vi "CopyIrAssetNodePropsToDevice.vi"(9 "Cameras":T12[](array[typedef]), 10 "AssetNodes":T1[](array[typedef]), 11 "DeviceModel in":T13) -> (3 "DeviceModel out":T13)   [LabVIEW 2017, in "ServerComm.lvlib"]
uses:
  <vilib>/addons/InsightCM/Devices/Shared/Common/ServerComm/ServerComm.lvlib
  <vilib>/addons/InsightCM/MessageBus/Base/controls/R2_DeviceModel.ctl
  <vilib>/addons/InsightCM/MessageBus/Base/controls/R2_Device.ctl
  <vilib>/addons/InsightCM/MessageBus/Base/controls/KeyValuePair.ctl
  <vilib>/addons/InsightCM/MessageBus/Base/controls/DeviceState.ctl
  <vilib>/addons/InsightCM/MessageBus/Base/controls/R2_DataGroup.ctl
  <vilib>/addons/InsightCM/MessageBus/Base/controls/OperatingState.ctl
  <vilib>/addons/InsightCM/MessageBus/Base/controls/Trigger.ctl
  <vilib>/addons/InsightCM/MessageBus/Base/controls/Condition.ctl
  <vilib>/addons/InsightCM/MessageBus/Base/controls/BurstModeTrigger.ctl
  <vilib>/addons/InsightCM/MessageBus/Base/controls/SensorGroup.ctl
  <vilib>/addons/InsightCM/MessageBus/Base/controls/Endpoint.ctl
  <vilib>/addons/InsightCM/MessageBus/Base/controls/WirelessChannel.ctl
  <vilib>/addons/InsightCM/MessageBus/Base/controls/R2_Channel.ctl
  <vilib>/addons/InsightCM/MessageBus/Base/controls/Metric.ctl
  <vilib>/addons/InsightCM/MessageBus/Base/controls/Tag.ctl
  <vilib>/addons/InsightCM/MessageBus/Base/controls/Camera.ctl
  <vilib>/addons/InsightCM/MessageBus/Base/controls/AssetNode.ctl
  <vilib>/addons/InsightCM/MessageBus/Base/controls/AssetState.ctl
  <vilib>/addons/InsightCM/MessageBus/Base/controls/TrendAlarmRule.ctl
  <vilib>/addons/InsightCM/MessageBus/Base/controls/TrendAlarmLevel.ctl
  <vilib>/addons/InsightCM/MessageBus/Base/controls/AlarmAction.ctl
  <vilib>/addons/InsightCM/MessageBus/Base/controls/AssetNodeReference.ctl
  <vilib>/addons/InsightCM/Utilities/PropertyHelpers/PropertyHelpers.lvlib
  <vilib>/addons/InsightCM/Utilities/DeviceModelHelpers/DeviceModelHelpers.lvlib
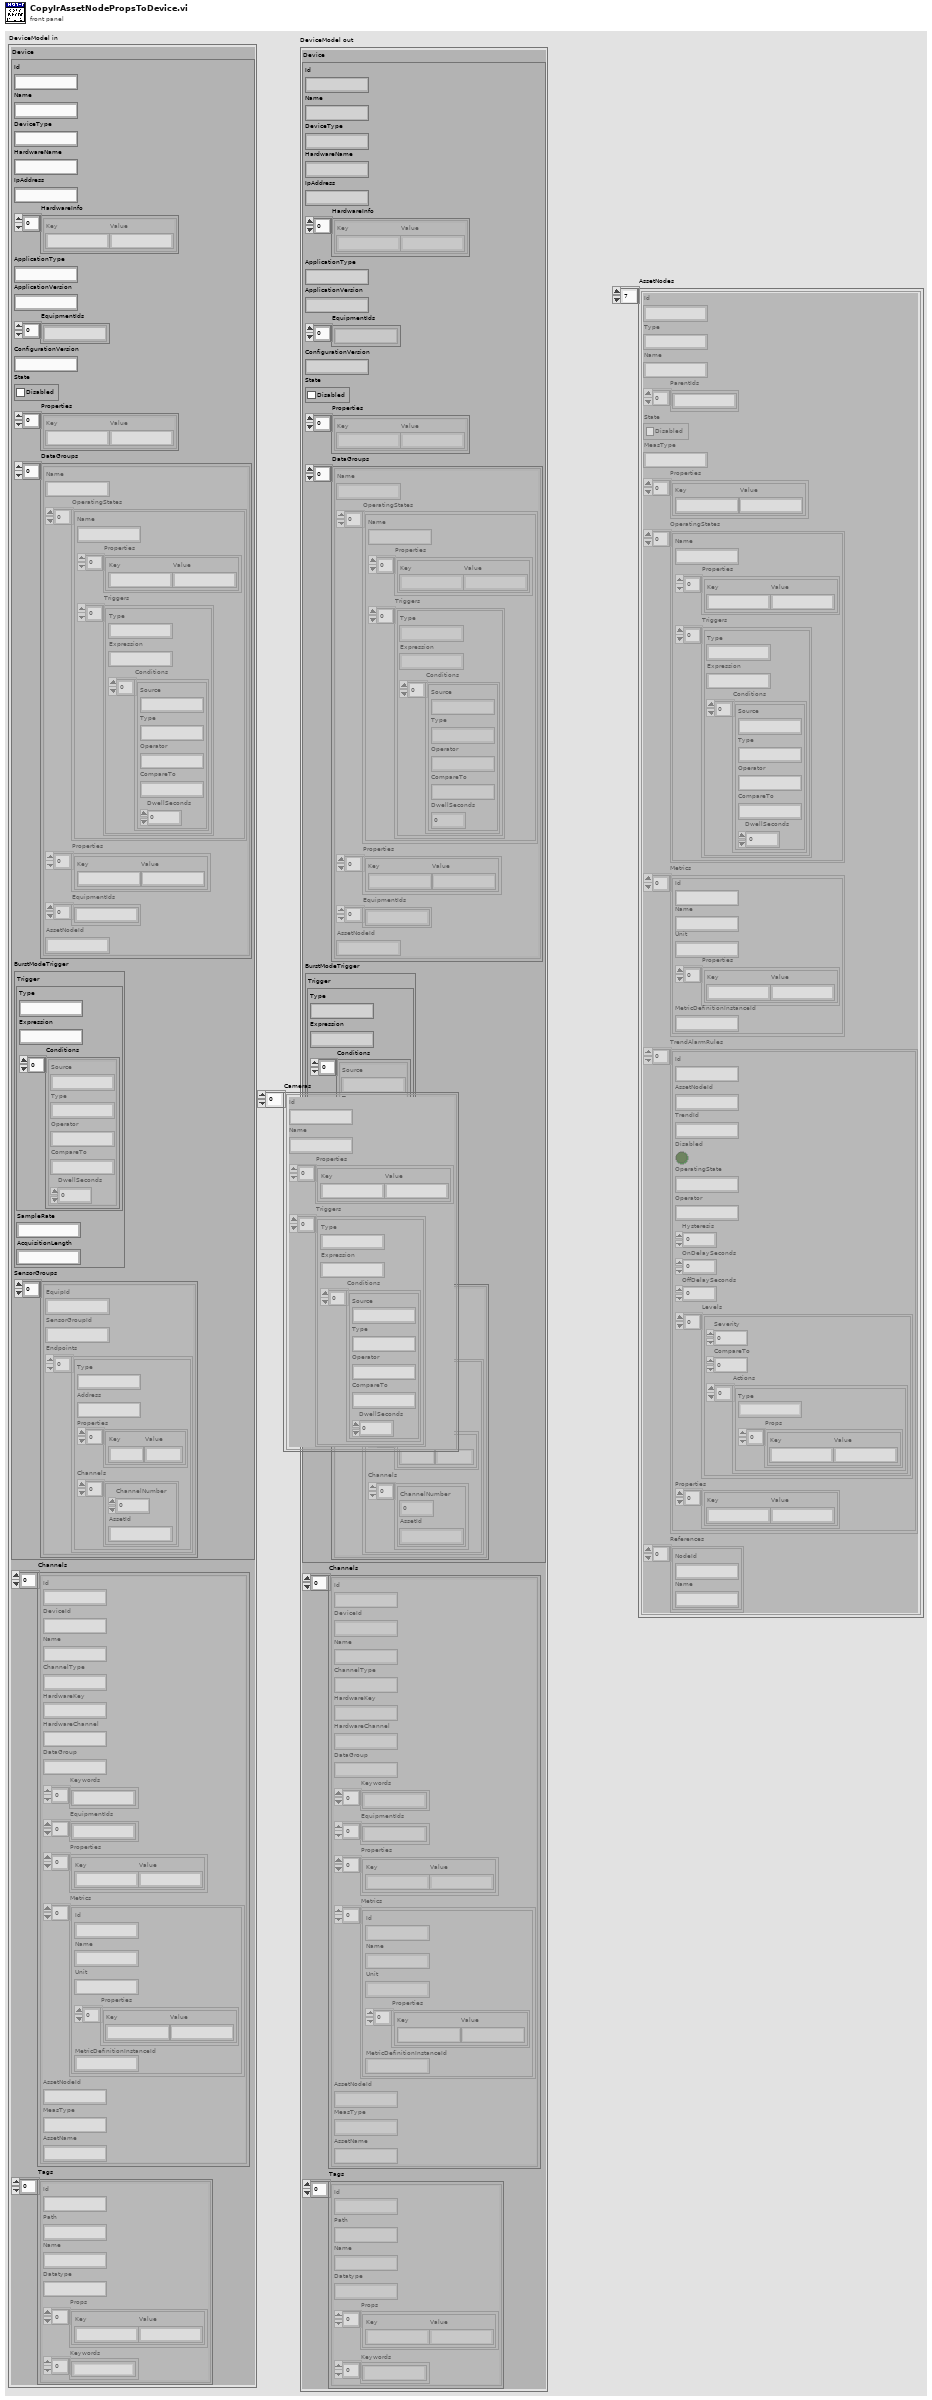
[diagram p1: front panel]
types:
  T1 = typedef "AssetNode.ctl" = cluster{"Id":string, "Type":string, "Name":string, "ParentIds":string[], "State":T2, "MeasType":string, "Properties":T3[], "OperatingStates":T4[], "Metrics":T7[], "TrendAlarmRules":T8[], "References":T11[]}
  T2 = typedef "AssetState.ctl" = cluster{"Disabled":bool}
  T3 = typedef "KeyValuePair.ctl" = cluster{"Key":string, "Value":string}
  T4 = typedef "OperatingState.ctl" = cluster{"Name":string, "Properties":T3[], "Triggers":T5[]}
  T5 = typedef "Trigger.ctl" = cluster{"Type":string, "Expression":string, "Conditions":T6[]}
  T6 = typedef "Condition.ctl" = cluster{"Source":string, "Type":string, "Operator":string, "CompareTo":string, "DwellSeconds":dbl}
  T7 = typedef "Metric.ctl" = cluster{"Id":string, "Name":string, "Unit":string, "Properties":T3[], "MetricDefinitionInstanceId":string}
  T8 = typedef "TrendAlarmRule.ctl" = cluster{"Id":string, "AssetNodeId":string, "TrendId":string, "Disabled":bool, "OperatingState":string, "Operator":string, "Hysteresis":dbl, "OnDelaySeconds":dbl, "OffDelaySeconds":dbl, "Levels":T9[], "Properties":T3[]}
  T9 = typedef "TrendAlarmLevel.ctl" = cluster{"Severity":i32, "CompareTo":dbl, "Actions":T10[]}
  T10 = typedef "AlarmAction.ctl" = cluster{"Type":string, "Props":T3[]}
  T11 = typedef "AssetNodeReference.ctl" = cluster{"NodeId":string, "Name":string}
  T12 = typedef "Camera.ctl" = cluster{"Id":string, "Name":string, "Properties":T3[], "Triggers":T5[]}
  T13 = typedef "R2_DeviceModel.ctl" = cluster{"Device":T14, "Channels":T21[], "Tags":T22[]}
  T14 = typedef "R2_Device.ctl" = cluster{"Id":string, "Name":string, "DeviceType":string, "HardwareName":string, "IpAddress":string, "HardwareInfo":T3[], "ApplicationType":string, "ApplicationVersion":string, "EquipmentIds":string[], "ConfigurationVersion":string, "State":T15, "Properties":T3[], "DataGroups":T16[], "BurstModeTrigger":T17, "SensorGroups":T18[]}
  T15 = typedef "DeviceState.ctl" = cluster{"Disabled":bool}
  T16 = typedef "R2_DataGroup.ctl" = cluster{"Name":string, "OperatingStates":T4[], "Properties":T3[], "EquipmentIds":string[], "AssetNodeId":string}
  T17 = typedef "BurstModeTrigger.ctl" = cluster{"Trigger":T5, "SampleRate":string, "AcquisitionLength":string}
  T18 = typedef "SensorGroup.ctl" = cluster{"EquipId":string, "SensorGroupId":string, "Endpoints":T19[]}
  T19 = typedef "Endpoint.ctl" = cluster{"Type":string, "Address":string, "Properties":T3[], "Channels":T20[]}
  T20 = typedef "WirelessChannel.ctl" = cluster{"ChannelNumber":i32, "AssetId":string}
  T21 = typedef "R2_Channel.ctl" = cluster{"Id":string, "DeviceId":string, "Name":string, "ChannelType":string, "HardwareKey":string, "HardwareChannel":string, "DataGroup":string, "Keywords":string[], "EquipmentIds":string[], "Properties":T3[], "Metrics":T7[], "AssetNodeId":string, "MeasType":string, "AssetName":string}
  T22 = typedef "Tag.ctl" = cluster{"Id":string, "Path":string, "Name":string, "Datatype":string, "Props":T3[], "Keywords":string[]}
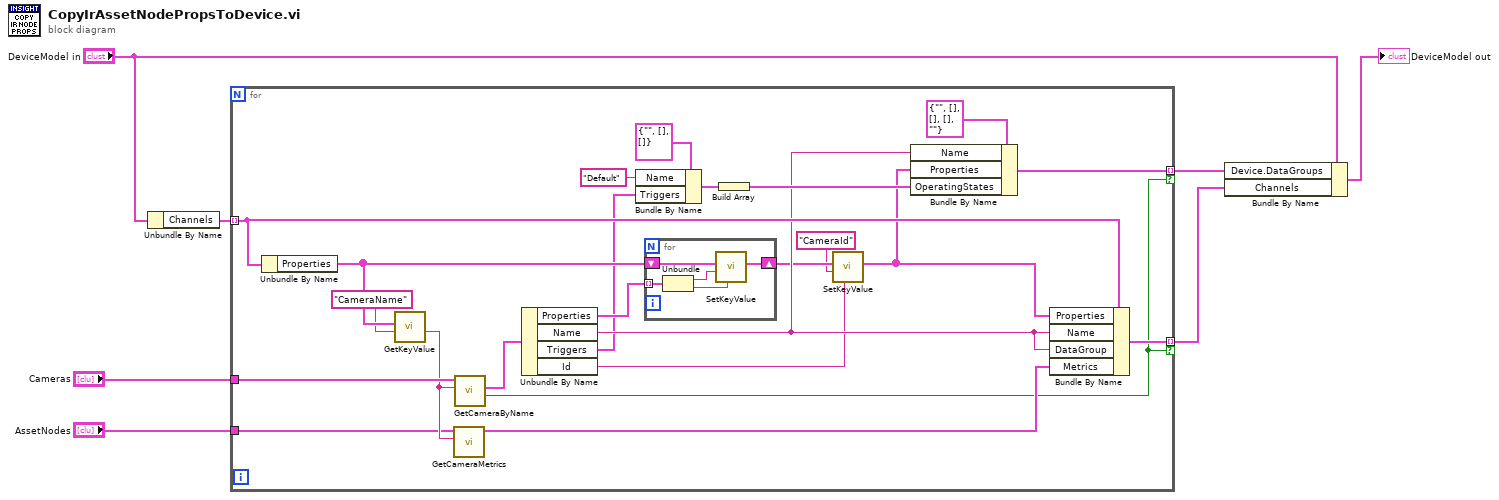
[diagram p0: block diagram]
diagram:
  n1 = Unbundle By Name("DeviceModel in") -> ("Channels"=w4:T21[])
  n2 = for {
    tunnel: [w30] -> w5 mode=indexing if=w8
    tunnel: w4 -> [w27] mode=indexing
    tunnel: [w28] -> w3 mode=indexing if=w8
    tunnel: "Cameras" -> [w24]
    tunnel: "AssetNodes" -> [w9]
    n3 = Unbundle By Name(w27) -> ("Properties"=w20:T3[])
    n4 = call <vilib>:"GetKeyValue.vi"("key"="CameraName", "key value pairs"=w20) -> ("value"=w10:string)  [unwired: 7 in, 2 out]
    n5 = call <vilib>:"GetCameraMetrics.vi"("camera name"=w10, "AssetNodes"=w9) -> ("mertics"=w11:T7[])  [unwired: 9 in]
    n6 = call <vilib>:"GetCameraByName.vi"("name"=w10, "cameras in"=w24) -> ("found"=w8:bool, "camera"=w25:T12)  [unwired: 7 in, 1 out]
    n7 = Unbundle By Name(w25) -> ("Properties"=w26:T3[], "Name"=w17:string, "Triggers"=w16:T5[], "Id"=w12:string)
    n8 = Bundle By Name(cluster=T4 {"Name"="", "Properties"=[], "Triggers"=[]} ("OperatingState 2"), "Name"="Default", "Triggers"=w16) -> (w22:T4)
    n9 = for {
      shift-right: [w33] -> w15
      shift-left: w20 -> [w34]
      tunnel: w26 -> [w35] mode=indexing
      n10 = Unbundle(w35) -> ("Key"=w32:string, "Value"=w31:string)
      n11 = call <vilib>:"SetKeyValue.vi"("value"=w31, "key"=w32, "key value pairs"=w34) -> ("key value pairs out"=w33:T3[])  [unwired: 8 in]
    }
    n12 = Build Array(w22) -> (w21:T4[])
    n13 = call <vilib>:"SetKeyValue.vi"("value"=w12, "key"="CameraId", "key value pairs"=w15) -> ("key value pairs out"=w14:T3[])  [unwired: 8 in]
    n14 = Bundle By Name(cluster=T16 {"Name"="", "OperatingStates"=[], "Properties"=[], "EquipmentIds"=[], "AssetNodeId"=""} ("output cluster"), "Name"=w17, "Properties"=w14, "OperatingStates"=w21) -> (w28:T16)
    n15 = Bundle By Name(cluster=w27, "Properties"=w14, "Name"=w17, "DataGroup"=w17, "Metrics"=w11) -> (w30:T21)
  }
  n16 = Bundle By Name(cluster="DeviceModel in", "Device.DataGroups"=w3, "Channels"=w5) -> (→"DeviceModel out":T13)
